vi "Main.vi"(11 "Module Admin":refnum<class "Delacor_lib_QMH_Module Admin.lvclass">) -> ()   [LabVIEW 2024, in "Auto Modo.lvlib"]
doc: "This template is based off of the Queued Message Handler design pattern and the Queued Message Handler project template that ships with LabVIEW.\n\nThe main difference is that the queue is private to this module and communication between modules is performed via Broadcast and Request events.\n\nRequest events are wrapped in public API methods and are handled in the Event Handling Loop (EHL) of this VI. Any module can register for Broadcast events sent by this module. The EHL generates messages based on user interface actions.\n\nThe Message Handling Loop (MHL) processes messages generated by the EHL, or by other messages. The messages are string values, so new messages can be added easily to the Message Cases case structure in the MHL. Each message cluster can also provide an optional value for Message Data, which is a variant that can be converted to whatever message-specific data is required.\n_____\nBased on DQMH Project Template 7.0.1.1316."
uses:
  Auto Modo.lvlib
  <vilib>/Delacor/Delacor QMH/Libraries/Module Admin_class/Delacor_lib_QMH_Module Admin.lvclass
  Sequencer Data Context.ctl
  Sequencer State.ctl
  Module Data--cluster.ctl
  Stop Sequence (Reply Payload)--cluster.ctl
  Start Sequence (Reply Payload)--cluster.ctl
  <vilib>/Delacor/Delacor QMH/Libraries/Message Queue_class/Delacor_lib_QMH_Message Queue.lvclass/Delacor_lib_QMH_Message Queue.ctl
  Stop Argument--cluster.ctl
  <vilib>/Delacor/Delacor QMH/Libraries/Module Admin_class/Delacor_lib_QMH_Module Admin.lvclass/Delacor_lib_QMH_Module Admin.ctl
  Check Idle State Argument--cluster.ctl
  Check Idle State (Reply Payload)--cluster.ctl
  <vilib>/Utility/miscctls.llb/LVPointTypeDef.ctl
  <vilib>/Delacor/Delacor QMH/Libraries/Message Queue_class/Delacor_lib_QMH_Enqueue Message (Single).vi
  <vilib>/Delacor/Delacor QMH/Libraries/Module Admin_class/Delacor_lib_QMH_Get External Launch.vi
  <vilib>/Delacor/Delacor QMH/Libraries/Message Queue_class/Delacor_lib_QMH_Message Queue.lvclass
  Hardware Controller/Hardware Controller.lvlib
  Logger/Logger.lvlib
panel:
  out "Sequencer Data Context":T1={"Sequencer State"=enum."Idle", "Event Timeout"=-1, "Current Index"=0, "Sequence Timeout"=0, "Turbine RPM Array"=[], "Pump RPM Array"=[], "Duration (Seconds) Array"=[], "Folder Path"=path ""}
  out "System State":map{string, dbl}(c390)
  out "error out":errorcluster
  out "Status":string
  in  "Simulate MHL Error":bool
  in  "Simulate EHL Error":bool
  # "Global Variable"
  # "This template is for the DQMH framework. See the block diagram for more information on how to use this template."
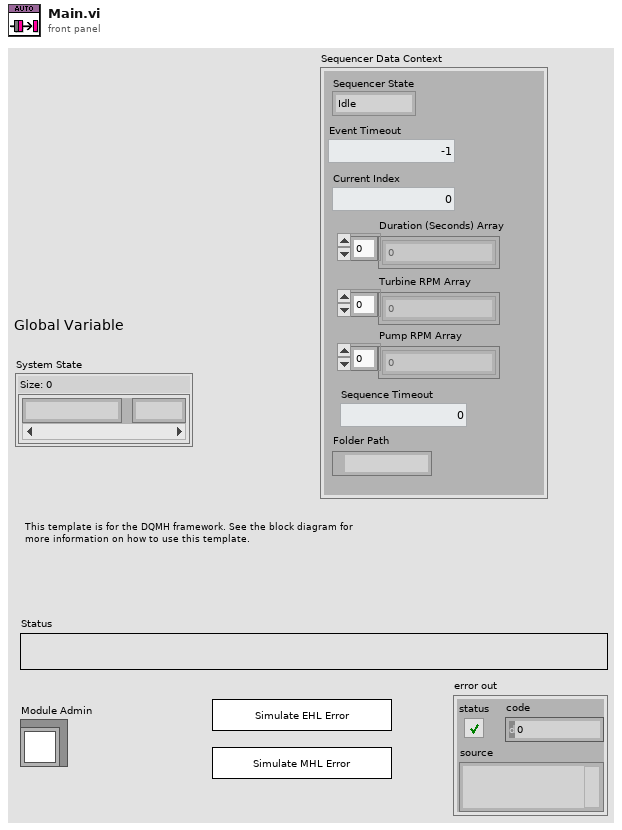
[diagram p1: front panel]
types:
  T1 = typedef "Auto Modo.lvlib/Sequencer Data Context.ctl" = cluster{"Sequencer State":T2, "Event Timeout":i32, "Current Index":i32, "Sequence Timeout":i32, "Turbine RPM Array":dbl[], "Pump RPM Array":dbl[], "Duration (Seconds) Array":dbl[], "Folder Path":path}
  T2 = typedef "Auto Modo.lvlib/Sequencer State.ctl" = enum16{"Idle", "Clear Drive Fault", "Check Drive Fault", "Set Ready to Switch ON", "Check Ready to Switch ON", "Enable Operation", "Check Enable Operation", "Set Drive RPM", "Check Drive RPM", "Next Drive RPM", "Final"}
  T3 = typedef "Auto Modo.lvlib/Request Events--cluster.ctl" = cluster{"Stop Module":refnum<user-event>, "Show Panel":refnum<user-event>, "Hide Panel":refnum<user-event>, "Get Module Execution Status":refnum<user-event>, "Show Diagram":refnum<user-event>, "Start Sequence":refnum<user-event>, "Stop Sequence":refnum<user-event>, "Check Idle State":refnum<user-event>}
  T4 = typedef "Hardware Controller.lvlib/Broadcast Events--cluster.ctl" = cluster{"Module Did Init":refnum<user-event>, "Status Updated":refnum<user-event>, "Error Reported":refnum<user-event>, "Module Did Stop":refnum<user-event>, "Update Module Execution Status":refnum<user-event>, "System State Updated":refnum<user-event>, "EtherCAT Data Updated":refnum<user-event>, "System Fault Updated":refnum<user-event>, "EtherCAT Connection Status Updated":refnum<user-event>, "HardwareController IOLink Data Updated":refnum<user-event>, "IOLink Connection Updated":refnum<user-event>, "HardwareController EtherCAT Data Updated":refnum<user-event>}
  T5 = typedef "Auto Modo.lvlib/Module Data--cluster.ctl" = cluster{"Status":string}
  T6 = typedef "Auto Modo.lvlib/Stop Sequence (Reply Payload)--cluster.ctl" = cluster{"error":errorcluster}
  T7 = typedef "Auto Modo.lvlib/Start Sequence (Reply Payload)--cluster.ctl" = cluster{"error":errorcluster}
  T8 = enum32{"invalid lock state", "Not Locked", "Locked (No Password)", "Password-protected"}
  T9 = typedef "Auto Modo.lvlib/Stop Argument--cluster.ctl" = cluster{"Origin":string, "Exit via Stop Module Req?":bool, "Wait for Module to stop?":bool}
  T10 = typedef "Auto Modo.lvlib/Check Idle State Argument--cluster.ctl" = cluster{"Wait Notifier":refnum<notifier>, "wait for reply":bool}
  T11 = typedef "LVPointTypeDef.ctl" = cluster{"Horizontal":i16, "Vertical":i16}
  T12 = enum32{"Invalid", "Standard", "Closed", "Hidden", "Minimized", "Maximized"}
  T13 = typedef "Auto Modo.lvlib/Check Idle State (Reply Payload)--cluster.ctl" = cluster{"Idle":bool, "error":errorcluster}
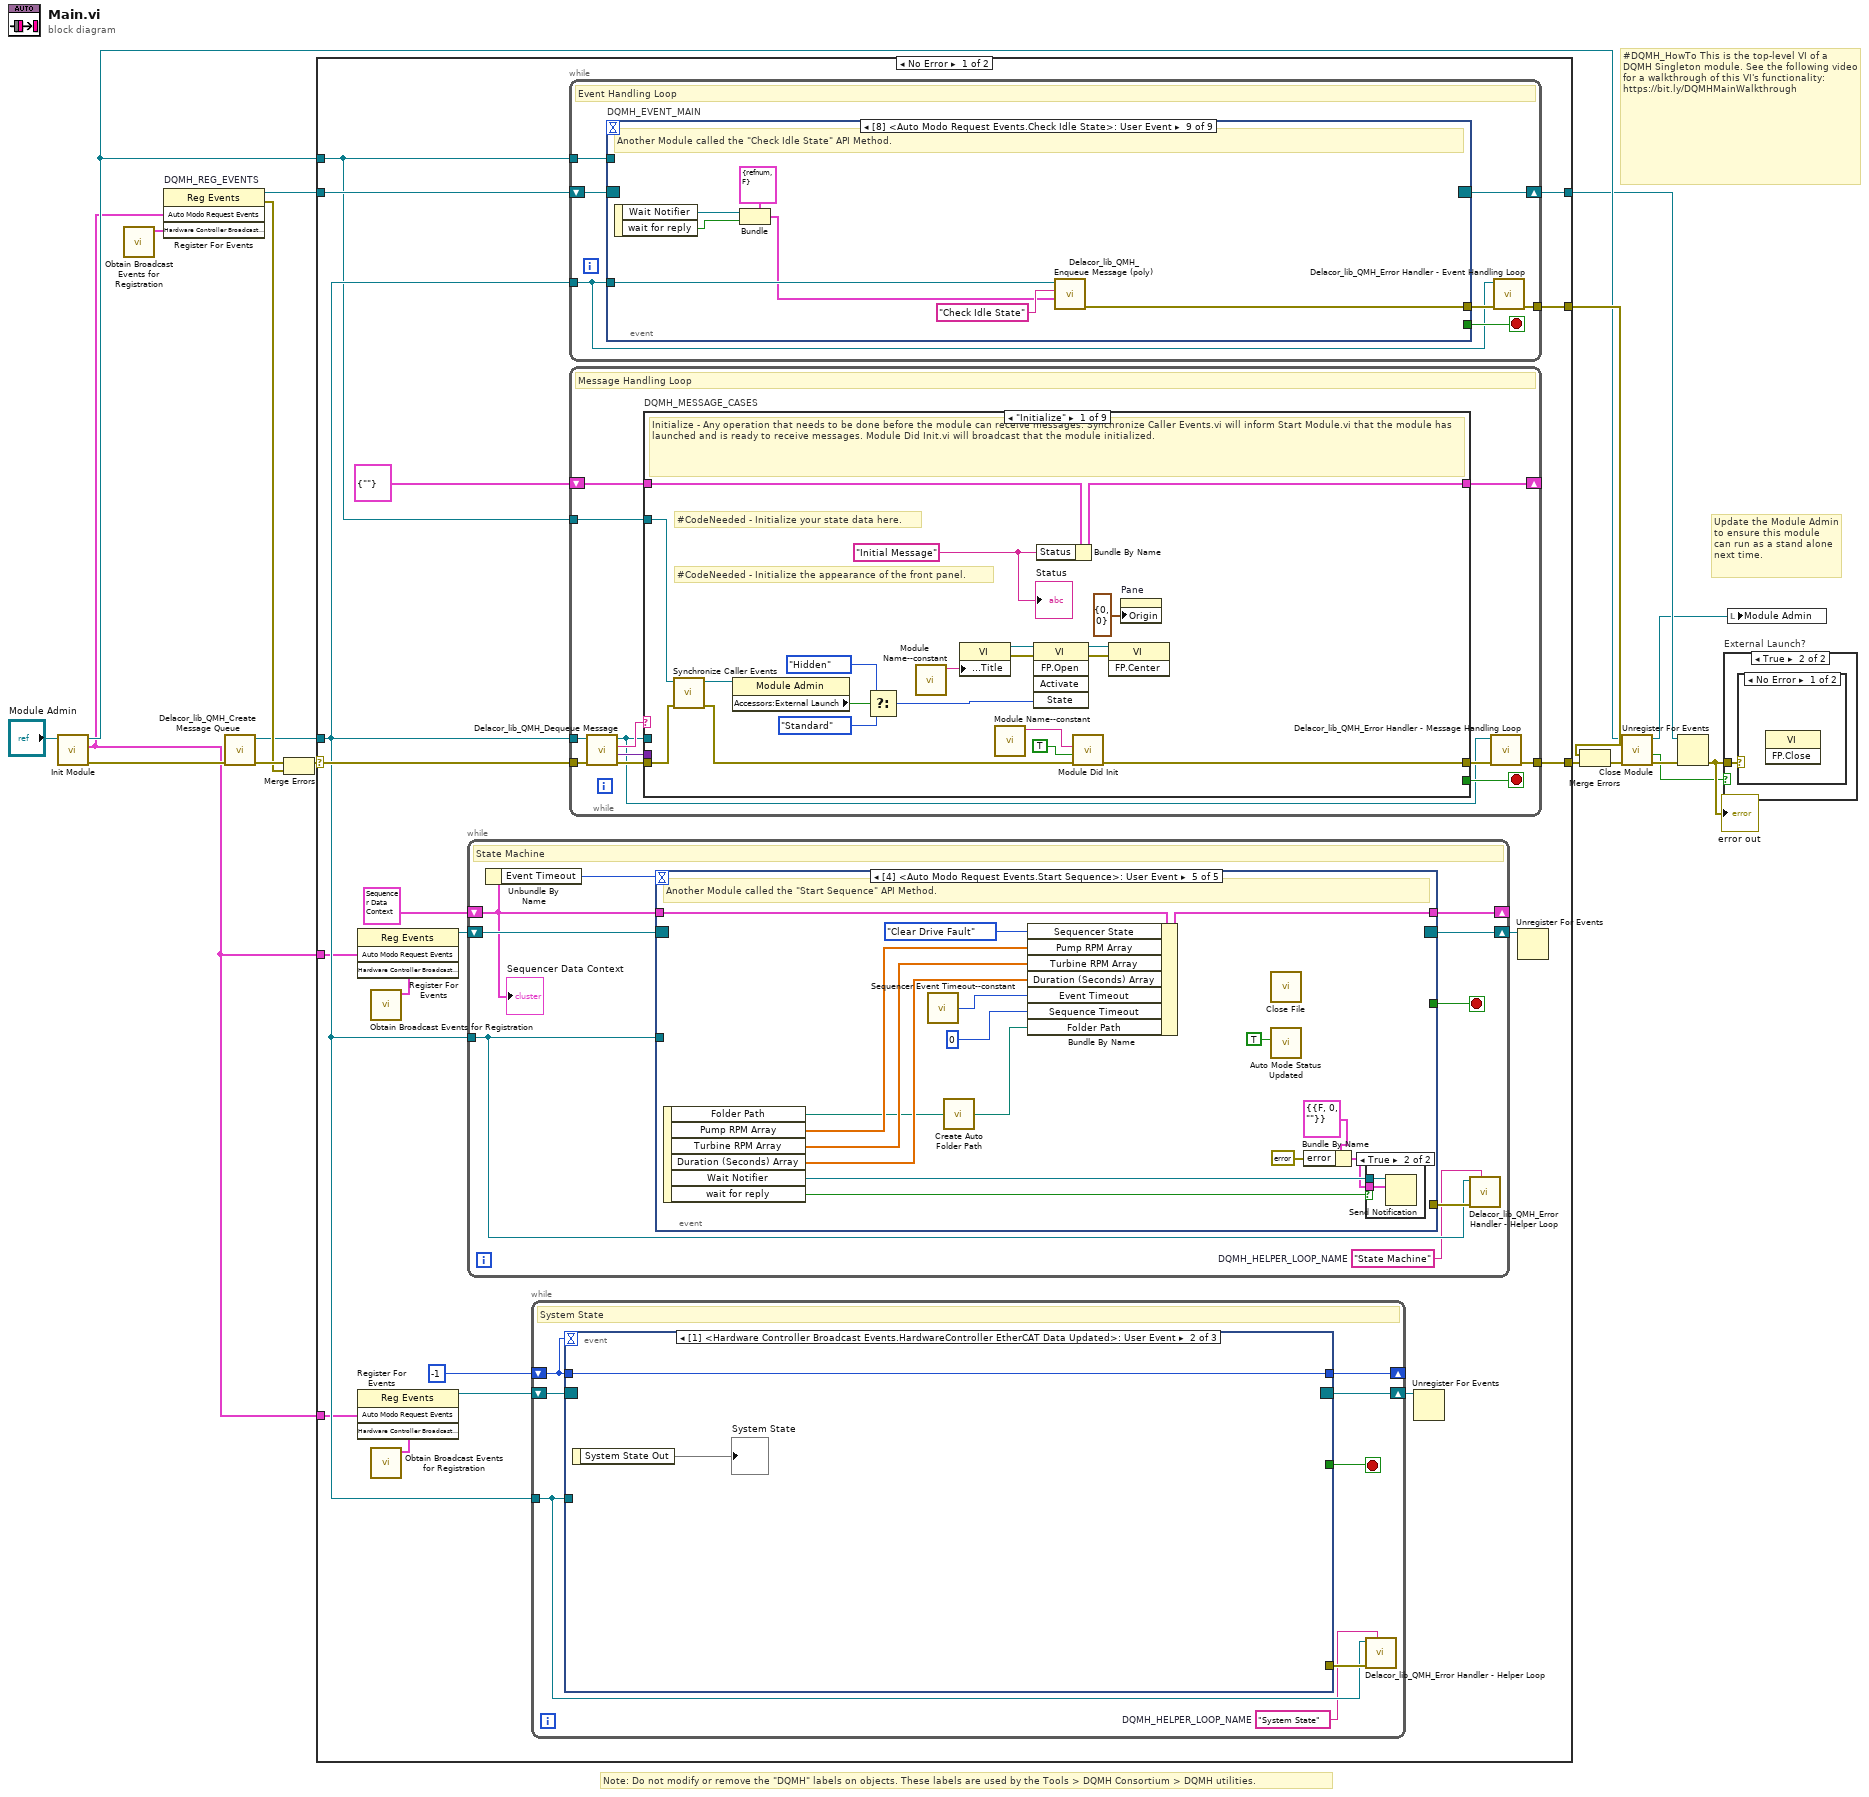
[diagram p0: block diagram]
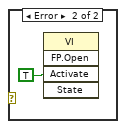
[diagram p3: hidden frame]
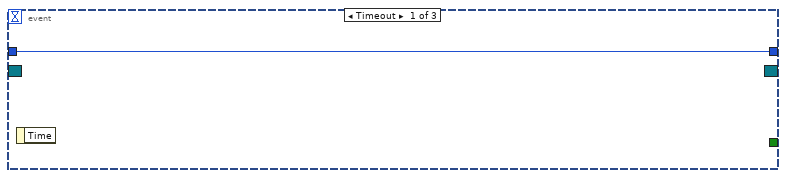
[diagram p4: hidden frame]
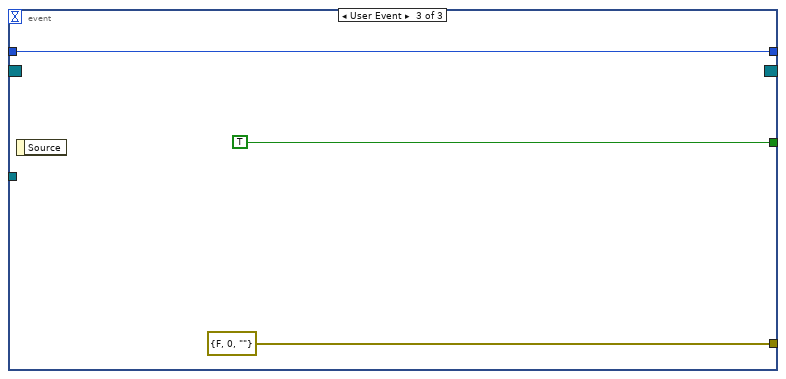
[diagram p5: hidden frame]
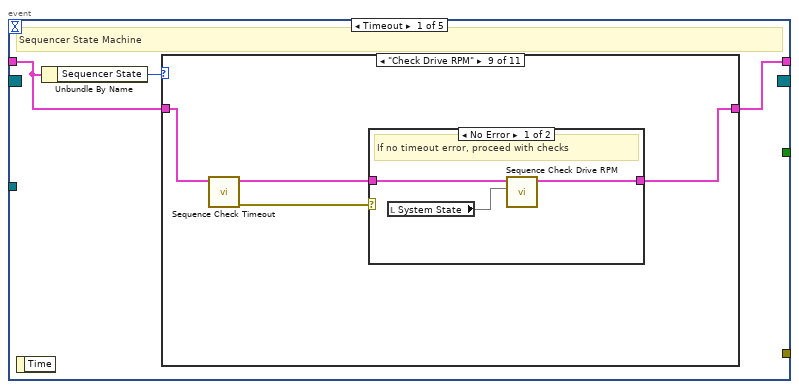
[diagram p6: hidden frame]
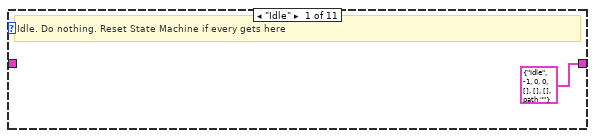
[diagram p7: hidden frame]
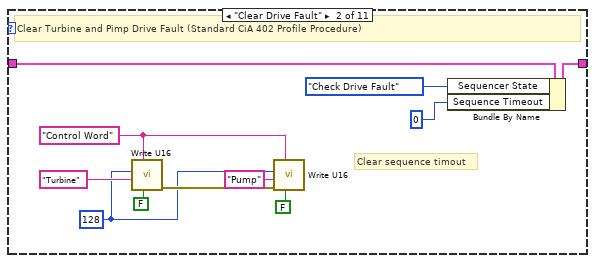
[diagram p8: hidden frame]
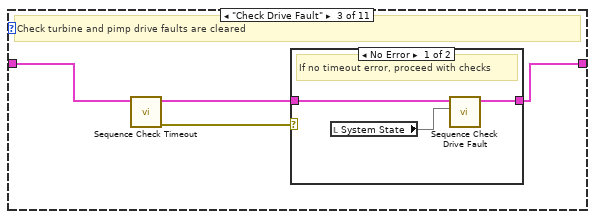
[diagram p9: hidden frame]
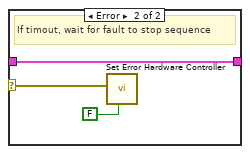
[diagram p10: hidden frame]
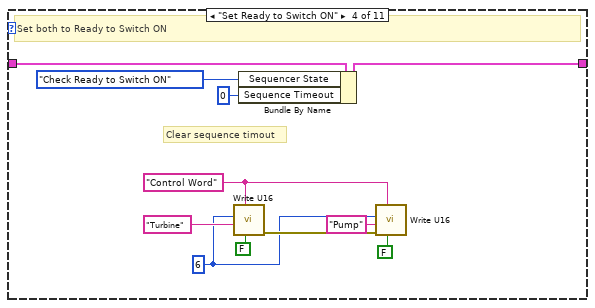
[diagram p11: hidden frame]
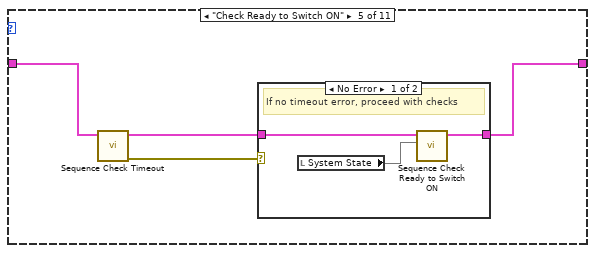
[diagram p12: hidden frame]
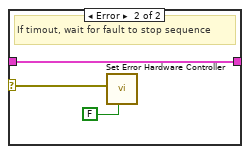
[diagram p13: hidden frame]
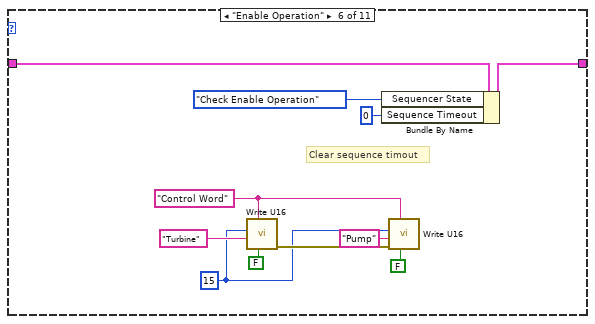
[diagram p14: hidden frame]
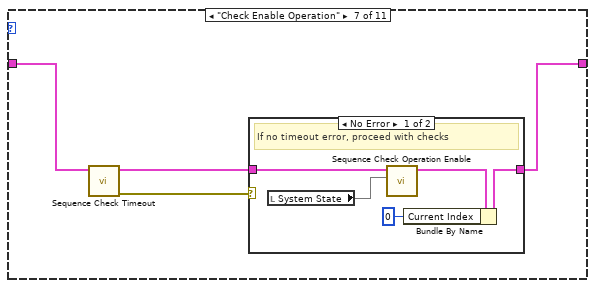
[diagram p15: hidden frame]
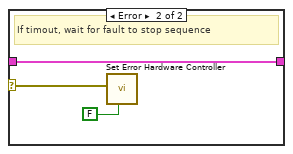
[diagram p16: hidden frame]
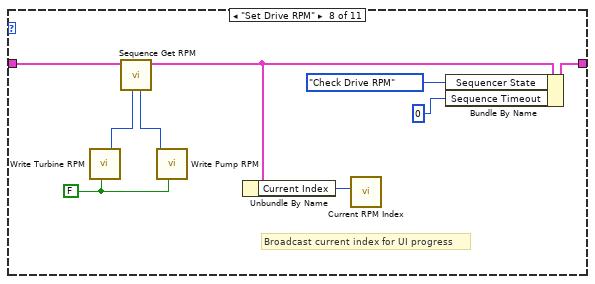
[diagram p17: hidden frame]
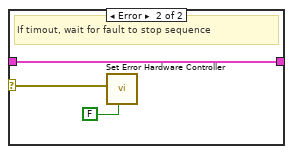
[diagram p18: hidden frame]
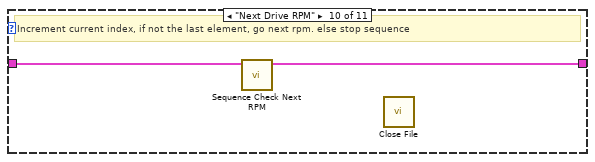
[diagram p19: hidden frame]
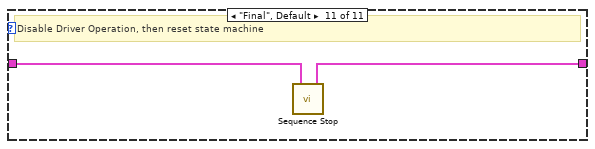
[diagram p20: hidden frame]
diagram:
  # "#DQMH_HowTo This is the top-level VI of a DQMH Singleton module. See the following video for a walkthrough of this VI's functionality: https://bit.ly/DQMHMainWalkthrough"
  # "Note: Do not modify or remove the \"DQMH\" labels on objects. These labels are used by the Tools > DQMH Consortium > DQMH utilities."
  # "Update the Module Admin to ensure this module can run as a stand alone next time."
  n1 = call "Init Module.vi"("Singleton Module Admin in"="Module Admin") -> ("error out"=w17:errorcluster, "Auto Modo Request Events"=w1:T3, "Singleton Module Admin out"=w9:refnum<class "Delacor_lib_QMH_Module Admin.lvclass">)  [unwired: 8 in]
  n2 = call "Obtain Broadcast Events for Registration.vi"() -> ("Hardware Controller Broadcast Events"=w2:T4)  [unwired: 9 in, 2 out]
  n3 = register-events "DQMH_REG_EVENTS"(w1, w2) -> (reference out=w7:refnum<event-registration>, error out=w10:errorcluster)  [unwired: 2 in]
  n4 = call <vilib>:"Delacor_lib_QMH_Create Message Queue.vi"("error in"=w17) -> ("error out"=w12:errorcluster, "Message Queue"=w6:refnum<class "Delacor_lib_QMH_Message Queue.lvclass">)  [unwired: 9 in]
  n5 = Merge Errors(w12, w10) -> (w11:errorcluster)
  n6 = case shown="No Error" w11 {
    selector: w11 -> [w34 w360]
    tunnel: [w36 w359] -> w18
    tunnel: [w33 w358] -> w8
    tunnel: w7 -> [w31 w358]
    tunnel: w6 -> [w30 w353]
    tunnel: [w35 _] -> w15
    tunnel: w9 -> [w29 w354]
    tunnel: w1 -> [w28 _]
    tunnel: w1 -> [w23 _]
    frame No Error {
      n7 = call "Obtain Broadcast Events for Registration.vi"() -> ("Hardware Controller Broadcast Events"=w24:T4)  [unwired: 9 in, 2 out]
      n8 = register-events ("DQMH_HELPER_REGFOREVENTS")(w28, w24) -> (reference out=w26:refnum<event-registration>)  [unwired: 2 in, 1 out]
      n9 = call "Obtain Broadcast Events for Registration.vi"() -> ("Hardware Controller Broadcast Events"=w19:T4)  [unwired: 9 in, 2 out]
      n10 = register-events ("DQMH_HELPER_REGFOREVENTS")(w23, w19) -> (reference out=w21:refnum<event-registration>)  [unwired: 2 in, 1 out]
      n11 = while "DQMH_HELPER_LOOP" {
        shift-right: [w59] -> _
        shift-left: T1 {"Sequencer State"=enum."Clear Drive Fault", "Event Timeout"=-1, "Current Index"=0, "Sequence Timeout"=-1, "Turbine RPM Array"=[], "Pump RPM Array"=[], "Duration (Seconds) Array"=[], "Folder Path"=path ""} ("Sequencer Data Context") -> [w52]
        shift-right: [w57] -> w27
        shift-left: w26 -> [w58]
        tunnel: w30 -> [w54]
        stop <- w56 stop-if-true
        w53 = "State Machine"  # DQMH_HELPER_LOOP_NAME
        # "State Machine"
        n12 = Unbundle By Name(w52) -> ("Event Timeout"=w51:i32)
        n13 = event "DQMH_HELPER_EVENT_STRUCTURE" shown="[4] <Auto Modo Request Events.Start Sequence>: User Event" {
          selector: w58 -> [_ _ _ _ _]
          dyn-events: [_ _ _ _ _] -> w57
          timeout: w51 -> [_ _ _ _ _]
          tunnel: w52 -> [w62 w152 w161 w163 w182]
          tunnel: [w60 w153 w162 w164 w177] -> w59
          tunnel: [_ _ _ TRUE _] -> w56
          tunnel: [_ _ _ errorcluster {"status"=FALSE, "code"=0, "source"=""} ("error constant") _] -> w55
          tunnel: w54 -> [_ _ _ _ _]
          event Timeout {
            # "Sequencer State Machine"
            n14 = event-data() -> ()  [unwired: 1 in, 1 out]
            n15 = Unbundle By Name(w62) -> ("Sequencer State"=w61:T2)
            n16 = case shown="\"Check Drive RPM\"" w61 {
              tunnel: w62 -> [_ w74 w77 w88 w97 w114 w118 w137 w139 w149 w150]
              tunnel: [T1 {"Sequencer State"=enum."Idle", "Event Timeout"=-1, "Current Index"=0, "Sequence Timeout"=0, "Turbine RPM Array"=[], "Pump RPM Array"=[], "Duration (Seconds) Array"=[], "Folder Path"=path ""} ("Sequencer Data Context") w66 w78 w87 w96 w113 w117 w136 w138 w148 w151] -> w60
              frame "Idle" {
                # "Idle. Do nothing. Reset State Machine if every gets here"
              }
              frame "Clear Drive Fault" {
                w73 = "Control Word" ("Variable")
                w68 = u16 128 ("Data")
                # "Clear sequence timout"
                # "Clear Turbine and Pimp Drive Fault (Standard CiA 402 Profile Procedure)"
                n17 = call "Write U16.vi"("wait for reply (T)"=FALSE, "Variable"=w73, "Drive"="Turbine", "Data"=w68) -> ("error out"=w71:errorcluster)  [unwired: 6 in, 1 out]
                n18 = call "Write U16.vi"("wait for reply (T)"=FALSE, "Variable"=w73, "error in"=w71, "Drive"="Pump", "Data"=w68) -> ()  [unwired: 5 in, 2 out]
                n19 = Bundle By Name(cluster=w74, "Sequencer State"=Sequencer_State."Check Drive Fault", "Sequence Timeout"=0) -> (w66:T1)
              }
              frame "Check Drive Fault" {
                # "Check turbine and pimp drive faults are cleared"
                n20 = call "Sequence Check Timeout.vi"("Sequencer Data Context IN"=w77) -> ("error out"=w75:errorcluster, "Sequencer Data Context OUT"=w76:T1)  [unwired: 9 in]
                n21 = case shown="No Error" w75 {
                  selector: w75 -> [_ w82]
                  tunnel: [w81 w84] -> w78
                  tunnel: w76 -> [w79 w84]
                  frame No Error {
                    # "If no timeout error, proceed with checks"
                    n22 = local read "System State"() -> (w80:map{string, dbl})
                    n23 = call "Sequence Check Drive Fault.vi"("System State"=w80, "Sequencer Data Context IN"=w79) -> ("Sequencer Data Context OUT"=w81:T1)  [unwired: 9 in]
                  }
                  frame Error {
                    # "If timout, wait for fault to stop sequence"
                    n24 = call "Set Error Hardware Controller.vi"("wait for reply (T)"=FALSE, "Error Cluster"=w82) -> ()  [unwired: 8 in, 2 out]
                  }
                }
              }
              frame "Set Ready to Switch ON" {
                w95 = "Control Word" ("Variable")
                w90 = u16 6 ("Data")
                # "Clear sequence timout"
                # "Set both to Ready to Switch ON"
                n25 = call "Write U16.vi"("wait for reply (T)"=FALSE, "Variable"=w95, "Drive"="Turbine", "Data"=w90) -> ("error out"=w93:errorcluster)  [unwired: 6 in, 1 out]
                n26 = Bundle By Name(cluster=w88, "Sequencer State"=Sequencer_State."Check Ready to Switch ON", "Sequence Timeout"=0) -> (w87:T1)
                n27 = call "Write U16.vi"("wait for reply (T)"=FALSE, "Variable"=w95, "error in"=w93, "Drive"="Pump", "Data"=w90) -> ()  [unwired: 5 in, 2 out]
              }
              frame "Check Ready to Switch ON" {
                n28 = call "Sequence Check Timeout.vi"("Sequencer Data Context IN"=w97) -> ("error out"=w98:errorcluster, "Sequencer Data Context OUT"=w99:T1)  [unwired: 9 in]
                n29 = case shown="No Error" w98 {
                  selector: w98 -> [_ w103]
                  tunnel: [w102 w105] -> w96
                  tunnel: w99 -> [w100 w105]
                  frame No Error {
                    # "If no timeout error, proceed with checks"
                    n30 = local read "System State"() -> (w101:map{string, dbl})
                    n31 = call "Sequence Check Ready to Switch ON.vi"("System State"=w101, "Sequencer Data Context IN"=w100) -> ("Sequencer Data Context OUT"=w102:T1)  [unwired: 9 in]
                  }
                  frame Error {
                    # "If timout, wait for fault to stop sequence"
                    n32 = call "Set Error Hardware Controller.vi"("wait for reply (T)"=FALSE, "Error Cluster"=w103) -> ()  [unwired: 8 in, 2 out]
                  }
                }
              }
              frame "Enable Operation" {
                w112 = "Control Word" ("Variable")
                w107 = u16 15 ("Data")
                # "Clear sequence timout"
                n33 = call "Write U16.vi"("wait for reply (T)"=FALSE, "Variable"=w112, "Drive"="Turbine", "Data"=w107) -> ("error out"=w110:errorcluster)  [unwired: 6 in, 1 out]
                n34 = Bundle By Name(cluster=w114, "Sequencer State"=Sequencer_State."Check Enable Operation", "Sequence Timeout"=0) -> (w113:T1)
                n35 = call "Write U16.vi"("wait for reply (T)"=FALSE, "Variable"=w112, "error in"=w110, "Drive"="Pump", "Data"=w107) -> ()  [unwired: 5 in, 2 out]
              }
              frame "Check Enable Operation" {
                n36 = call "Sequence Check Timeout.vi"("Sequencer Data Context IN"=w118) -> ("error out"=w119:errorcluster, "Sequencer Data Context OUT"=w120:T1)  [unwired: 9 in]
                n37 = case shown="No Error" w119 {
                  selector: w119 -> [_ w126]
                  tunnel: [w122 w128] -> w117
                  tunnel: w120 -> [w123 w128]
                  frame No Error {
                    # "If no timeout error, proceed with checks"
                    n38 = local read "System State"() -> (w124:map{string, dbl})
                    n39 = call "Sequence Check Operation Enable.vi"("System State"=w124, "Sequencer Data Context IN"=w123) -> ("Sequencer Data Context OUT"=w125:T1)  [unwired: 9 in]
                    n40 = Bundle By Name(cluster=w125, "Current Index"=0) -> (w122:T1)
                  }
                  frame Error {
                    # "If timout, wait for fault to stop sequence"
                    n41 = call "Set Error Hardware Controller.vi"("wait for reply (T)"=FALSE, "Error Cluster"=w126) -> ()  [unwired: 8 in, 2 out]
                  }
                }
              }
              frame "Set Drive RPM" {
                w129 = FALSE ("wait for reply (T)")
                # "Broadcast current index for UI progress"
                n42 = call "Sequence Get RPM.vi"("Sequencer Data Context IN"=w137) -> ("Sequencer Data Context OUT"=w133:T1, "Pump RPM"=w130:i16, "Turbine RPM"=w131:i16)  [unwired: 8 in]
                n43 = call "Write Turbine RPM.vi"("wait for reply (T)"=w129, "RPM"=w131) -> ()  [unwired: 8 in, 2 out]
                n44 = call "Write Pump RPM.vi"("wait for reply (T)"=w129, "RPM"=w130) -> ()  [unwired: 8 in, 2 out]
                n45 = Unbundle By Name(w133) -> ("Current Index"=w132:i32)
                n46 = call "Current RPM Index.vi"("Current Index"=w132) -> ()  [unwired: 10 in, 1 out]
                n47 = Bundle By Name(cluster=w133, "Sequencer State"=Sequencer_State."Check Drive RPM", "Sequence Timeout"=0) -> (w136:T1)
              }
              frame "Check Drive RPM" {
                n48 = call "Sequence Check Timeout.vi"("Sequencer Data Context IN"=w139) -> ("error out"=w140:errorcluster, "Sequencer Data Context OUT"=w141:T1)  [unwired: 9 in]
                n49 = case shown="No Error" w140 {
                  selector: w140 -> [_ w145]
                  tunnel: [w144 w147] -> w138
                  tunnel: w141 -> [w142 w147]
                  frame No Error {
                    # "If no timeout error, proceed with checks"
                    n50 = local read "System State"() -> (w143:map{string, dbl})
                    n51 = call "Sequence Check Drive RPM.vi"("System State"=w143, "Sequencer Data Context IN"=w142) -> ("Sequencer Data Context OUT"=w144:T1)  [unwired: 9 in]
                  }
                  frame Error {
                    # "If timout, wait for fault to stop sequence"
                    n52 = call "Set Error Hardware Controller.vi"("wait for reply (T)"=FALSE, "Error Cluster"=w145) -> ()  [unwired: 8 in, 2 out]
                  }
                }
              }
              frame "Next Drive RPM" {
                # "Increment current index, if not the last element, go next rpm. else stop sequence"
                n53 = call "Sequence Check Next RPM.vi"("Sequencer Data Context IN"=w149) -> ("Sequencer Data Context OUT"=w148:T1)  [unwired: 10 in]
                n54 = call "Close File.vi"() -> ()  [unwired: 9 in, 3 out]
              }
              frame "Final", Default {
                # "Disable Driver Operation, then reset state machine"
                n55 = call "Sequence Stop.vi"("Sequencer Data Context IN"=w150) -> ("Sequencer Data Context OUT"=w151:T1)
              }
            }
          }
          event User Event {
            # "Another Module called the \"Stop Sequence\" API Method."
            n56 = event-data() -> ("Wait Notifier"=w156:refnum<notifier>, "wait for reply"=w155:bool)  [unwired: 1 in]
            n57 = call "Sequence Stop.vi"("Sequencer Data Context IN"=w152) -> ("Sequencer Data Context OUT"=w153:T1)
            n58 = Bundle By Name(cluster=T6 {"error"={"status"=FALSE, "code"=0, "source"=""}} ("Stop Sequence (Reply Payload)"), "error"=errorcluster {"status"=FALSE, "code"=0, "source"=""}) -> (w158:T6)
            n59 = case "DQMH_FIRE_NOTIFIER" shown="True" w155 {
              tunnel: w156 -> [_ w160]
              tunnel: w158 -> [_ w159]
              frame False {
              }
              frame True {
                n60 = Send Notification(notification=w159, notifier=w160) -> ()  [unwired: 1 in, 2 out]
              }
            }
          }
          event User Event {
            n61 = event-data() -> ()  [unwired: 1 in, 1 out]
            n62 = call "Sequence Stop.vi"("Sequencer Data Context IN"=w161) -> ("Sequencer Data Context OUT"=w162:T1)
          }
          event User Event {
            n63 = event-data() -> ()  [unwired: 1 in, 1 out]
            n64 = call "Sequence Stop.vi"("Sequencer Data Context IN"=w163) -> ("Sequencer Data Context OUT"=w164:T1)
          }
          event User Event {
            # "Another Module called the \"Start Sequence\" API Method."
            n65 = event-data() -> ("Folder Path"=w169:path, "Pump RPM Array"=w172:dbl[], "Turbine RPM Array"=w171:dbl[], "Duration (Seconds) Array"=w170:dbl[], "Wait Notifier"=w181:refnum<notifier>, "wait for reply"=w180:bool)  [unwired: 1 in]
            n66 = call "Sequencer Event Timeout--constant.vi"() -> ("Event Timeout (ms)"=w174:i32)  [unwired: 1 in]
            n67 = call "Create Auto Folder Path.vi"("Parent Folder Path"=w169) -> ("Auto Folder Path"=w168:path)
            n68 = Bundle By Name(cluster=w182, "Sequencer State"=Sequencer_State."Clear Drive Fault", "Pump RPM Array"=w172, "Turbine RPM Array"=w171, "Duration (Seconds) Array"=w170, "Event Timeout"=w174, "Sequence Timeout"=0, "Folder Path"=w168) -> (w177:T1)
            n69 = call "Close File.vi"() -> ()  [unwired: 9 in, 3 out]
            n70 = call "Auto Mode Status Updated.vi"("Auto Mode?"=TRUE) -> ()  [unwired: 10 in, 1 out]
            n71 = Bundle By Name(cluster=T7 {"error"={"status"=FALSE, "code"=0, "source"=""}} ("Start Sequence (Reply Payload)"), "error"=errorcluster {"status"=FALSE, "code"=0, "source"=""}) -> (w179:T7)
            n72 = case "DQMH_FIRE_NOTIFIER" shown="True" w180 {
              tunnel: w181 -> [_ w184]
              tunnel: w179 -> [_ w183]
              frame False {
              }
              frame True {
                n73 = Send Notification(notification=w183, notifier=w184) -> ()  [unwired: 1 in, 2 out]
              }
            }
          }
        }
        n74 = call-dynamic "Delacor_lib_QMH_Error Handler - Helper Loop.vi"("Error Debug"=w53, "error in"=w55, "Message Queue in"=w54) -> ()  [unwired: 7 in, 2 out]
        "Sequencer Data Context" <- w52
      }
      n75 = while "DQMH_HELPER_LOOP" {
        shift-right: [w44] -> _
        shift-left: -1 -> [w43]
        shift-right: [w41] -> w22
        shift-left: w21 -> [w42]
        tunnel: w30 -> [w38]
        stop <- w40 stop-if-true
        w37 = "System State"  # DQMH_HELPER_LOOP_NAME
        # "System State"
        n76 = event "DQMH_HELPER_EVENT_STRUCTURE" shown="[1] <Hardware Controller Broadcast Events.HardwareController EtherCAT Data Updated>: User Event" {
          selector: w42 -> [_ _ _]
          dyn-events: [_ _ _] -> w41
          timeout: w43 -> [_ _ _]
          tunnel: w43 -> [w45 w47 w50]
          tunnel: [w45 w47 w50] -> w44
          tunnel: [_ _ TRUE] -> w40
          tunnel: [_ _ errorcluster {"status"=FALSE, "code"=0, "source"=""} ("error constant")] -> w39
          tunnel: w38 -> [_ _ _]
          event Timeout {
            n77 = event-data() -> ()  [unwired: 1 in, 1 out]
          }
          event User Event {
            n78 = event-data() -> ("System State Out"=→"System State":map{string, dbl})  [unwired: 1 in]
          }
          event User Event {
            n79 = event-data() -> ()  [unwired: 1 in, 1 out]
          }
        }
        n80 = call-dynamic "Delacor_lib_QMH_Error Handler - Helper Loop.vi"("Error Debug"=w37, "error in"=w39, "Message Queue in"=w38) -> ()  [unwired: 7 in, 2 out]
      }
      n81 = while {
        tunnel: w30 -> [w185]
        shift-right: [w188] -> w33
        shift-left: w31 -> [w189]
        tunnel: [w190] -> w35
        tunnel: w29 -> [w186]
        stop <- w187 stop-if-true
        # "Event Handling Loop"
        n82 = event "DQMH_EVENT_MAIN" shown="[8] <Auto Modo Request Events.Check Idle State>: User Event" {
          selector: w189 -> [_ _ _ _ _ _ _ _ _]
          dyn-events: [_ _ _ _ _ _ _ _ _] -> w188
          timeout: _ -> [_ _ _ _ _ _ _ _ _]
          tunnel: [_ _ _ _ _ _ TRUE ("Discard?") _ _] -> w187
          tunnel: w185 -> [_ w199 _ _ _ _ w223 w230 w246]
          tunnel: [w197 w200 _ _ w206 _ w226 w232 w240] -> w191
          tunnel: w186 -> [_ _ _ _ _ _ _ w229 _]
          event "Simulate EHL Error": Value Change {
            # "#DQMH_HowTo The 'Simulate EHL Error' button  illustrates how the EHL handles errors. This event is instructional in nature and can be removed."
            # "This case simulates an error being generated by the EHL"
            n83 = event-data() -> ()  [unwired: 1 in, 1 out]
            n84 = call "Module Name--constant.vi"() -> ("Module Name"=w194:string)  [unwired: 11 in]
            n85 = Format Into String(format string="Simulated error originating at Event Handling Loop in %s", w194) -> (resulting string=w195:string)  [unwired: 2 in, 1 out]
            n86 = call <vilib>:"Error Cluster From Error Code.vi"("show call chain? (False)"=TRUE, "error message (\"\")"=w195, "error code (0)"=5000) -> ("error out"=w197:errorcluster)  [unwired: 6 in]
          }
          event "Simulate MHL Error": Value Change {
            # "#DQMH_HowTo The 'Simulate MHL Error' button  illustrates how the MHL handles errors. This event is instructional in nature and can be removed."
            # "This case simulates an error being generated by the MHL"
            n87 = event-data() -> ()  [unwired: 1 in, 1 out]
            n88 = call-poly <vilib>:"Delacor_lib_QMH_Enqueue Message (poly).vi"("Message"="Simulate MHL Error", "Message Queue in"=w199) -> ("error out"=w200:errorcluster)  [unwired: 8 in, 1 out]
          }
          event User Event {
            # "Show the panel of this VI, and send a status updated message to let listeners know."
            # "Another Module called the \"Show Panel\" API Method."
            n89 = event-data() -> ()  [unwired: 1 in, 1 out]
            n90 = control-ref of="This VI"() -> (w202:refnum<vi>)
            n91 = call "Open VI Panel.vi"("VI"=w202) -> ()  [unwired: 10 in, 1 out]
            n92 = call "Status Updated.vi"("Status"="Panel shown." ("format string")) -> ()  [unwired: 10 in, 1 out]
          }
          event User Event {
            # "Hide the panel of this VI, and send a status updated message to let listeners know."
            # "Another Module called the \"Hide Panel\" API Method."
            n93 = event-data() -> ()  [unwired: 1 in, 1 out]
            n94 = control-ref of="This VI"() -> (w204:refnum<vi>)
            n95 = call "Hide VI Panel.vi"("VI"=w204) -> ()  [unwired: 10 in, 1 out]
            n96 = call "Status Updated.vi"("Status"="Panel hidden." ("format string")) -> ()  [unwired: 10 in, 1 out]
          }
          event User Event {
            # "Another Module called the \"Get Module Execution Status\" API Method."
            n97 = event-data() -> ()  [unwired: 1 in, 1 out]
            n98 = call "Update Module Execution Status.vi"("Running?"=TRUE) -> ("error out"=w206:errorcluster)  [unwired: 10 in]
          }
          event User Event {
            # "Another Module called the \"Show Diagram\" API Method. This event is used for debugging."
            n99 = event-data() -> ()  [unwired: 1 in, 1 out]
            n100 = disable-structure shown="RUN_TIME_ENGINE==False" {
              frame condition #0 (active) {
                # "functionality not available in exe"
                n101 = invoke on="Invoke Node" class="VI" method="Lock State.Get"() -> (error out=w212:errorcluster, "Get Lock State"=w211:T8, "pwd in cache"=w208:bool)  [unwired: 4 in, 1 out]
                n102 = Equal?(x=T8."Password-protected", y=w211) -> (x = y?=w209:bool)
                n103 = Compound Arithmetic op=AND(w209, invert w208) -> (w207:bool)
                n104 = case shown="False" w207 {
                  tunnel: w212 -> [w215 _]
                  frame False {
                    n105 = property on="Property Node" class="VI"(error in=w215, "BDWin.Open"=TRUE ("Block Diagram Window:Open")) -> ()  [unwired: 1 in, 2 out]
                    n106 = call "Status Updated.vi"("Status"="Block Diagram shown." ("format string")) -> ()  [unwired: 10 in, 1 out]
                  }
                  frame True {
                    # "Password-protected VI, and the password is not in the cache. Do not show the diagram."
                  }
                }
              }
              frame condition #1 {
              }
            }
          }
          event User Event {
            # "The Stop Module Event can get fired from the Exit message in the MHL. The queue gets destroyed in that case. If the queue no longer exists, the Enqueue Exit as a priority message will return error 1. It is safe to ignore, because the module is already exiting."
            # "Another Module called the \"Stop Module\" API Method  or the Message Handling Loop below."
            n107 = event-data() -> ("Origin"=w222:string, "Exit via Stop Module Req?"=w218:bool, "Wait for Module to stop?"=w217:bool)  [unwired: 1 in]
            n108 = local write "Status"(w222) -> ()
            n109 = Bundle By Name(cluster=T9 {"Origin"="", "Exit via Stop Module Req?"=FALSE, "Wait for Module to stop?"=FALSE} ("Stop Argument"), "Exit via Stop Module Req?"=w218, "Wait for Module to stop?"=w217) -> (w216:T9)
            n110 = call-poly <vilib>:"Delacor_lib_QMH_Enqueue Message (poly).vi"("Priority Message? (F)"=TRUE, "Message Data"=w216, "Message"="Exit", "Message Queue in"=w223) -> ("error out"=w227:errorcluster)  [unwired: 6 in, 1 out]
            n111 = call <vilib>:"Clear Errors.vi"("error in (no error)"=w227, "specific error code to clear (0: all)"=1) -> ("error out"=w226:errorcluster)  [unwired: 4 in, 1 out]
          }
          event Panel Close? {
            w231 = TRUE  # Discard the event, the MHL is responsible for closing and stopping this VI.
            # "Hide the panel or send the 'Exit' message if the user clicks the 'X' on the module main VI panel."
            n112 = event-data() -> ()  [unwired: 1 in, 1 out]
            n113 = property on="Property Node" class="Module Admin"(reference=w229) -> ("Accessors:External Launch"=w228:bool)  [unwired: 1 in, 2 out]
            n114 = case shown="True" w228 {
              tunnel: w230 -> [_ w238]
              tunnel: [_ w239] -> w232
              frame True {
                # "If externally launched, clicking the 'X' hides the panel, but doesn't close it."
                n115 = control-ref of="This VI"() -> (w235:refnum<vi>)
                n116 = call "Hide VI Panel.vi"("VI"=w235) -> ("error out"=w233:errorcluster)  [unwired: 10 in]
                n117 = call "Status Updated.vi"("error in"=w233, "Status"="Panel hidden." ("format string")) -> ()  [unwired: 9 in, 1 out]
              }
              frame False {
                # "If run as a stand-alone VI, clicking the panel 'X' stops the VI."
                n118 = call-poly <vilib>:"Delacor_lib_QMH_Enqueue Message (poly).vi"("Priority Message? (F)"=TRUE, "Message"="Exit", "Message Queue in"=w238) -> ("error out"=w239:errorcluster)  [unwired: 7 in, 1 out]
              }
            }
            n119 = event-data ("Event Filter Node")("Discard?"=w231) -> ()  [unwired: 1 in, 1 out]
          }
          event User Event {
            # "Another Module called the \"Check Idle State\" API Method."
            n120 = event-data() -> ("Wait Notifier"=w242:refnum<notifier>, "wait for reply"=w241:bool)  [unwired: 1 in]
            n121 = Bundle(cluster=T10 {"Wait Notifier"=refnum, "wait for reply"=FALSE} ("Check Idle State Argument"), "Wait Notifier"=w242, "wait for reply"=w241) -> (w243:T10)
            n122 = call-poly <vilib>:"Delacor_lib_QMH_Enqueue Message (poly).vi"("Message Data"=w243, "Message"="Check Idle State", "Message Queue in"=w246) -> ("error out"=w240:errorcluster)  [unwired: 7 in, 1 out]
          }
        }
        n123 = call-dynamic "Delacor_lib_QMH_Error Handler - Event Handling Loop.vi"("error in"=w191, "Message Queue in"=w185) -> ("dup error in"=w190:errorcluster)  [unwired: 8 in, 1 out]
      }
      n124 = while {
        tunnel: w30 -> [w247]
        shift-right: [w255] -> _
        shift-left: T5 {"Status"=""} ("Data Cluster") -> [w256]
        tunnel: w34 -> [w258]
        tunnel: [w250] -> w36
        tunnel: w29 -> [w251]
        stop <- w254 stop-if-true
        # "Message Handling Loop"
        n125 = call-dynamic "Delacor_lib_QMH_Dequeue Message.vi"("error in"=w258, "Message Queue in"=w247) -> ("error out"=w257:errorcluster, "Message Data"=w252:variant, "Message"=w253:string, "Message Queue out"=w248:refnum<class "Delacor_lib_QMH_Message Queue.lvclass">)  [unwired: 6 in]
        n126 = case "DQMH_MESSAGE_CASES" shown="\"Initialize\"" w253 {
          selector: w253 -> [_ _ _ _ _ _ _ _ w348]
          tunnel: w248 -> [_ _ _ _ _ _ w314 w336 _]
          tunnel: w257 -> [w276 w280 w294 w299 w301 w310 w321 w342 w351]
          tunnel: [w274 w280 w292 w298 w301 w309 w317 w337 w352] -> w249
          tunnel: w256 -> [w265 w279 w293 w297 w300 w307 w316 w335 w349]
          tunnel: [w264 w279 w293 w297 w300 w307 w316 w335 w349] -> w255
          tunnel: [_ _ _ _ _ _ _ w334 _] -> w254
          tunnel: w252 -> [_ _ w291 _ _ _ w315 w333 _]
          tunnel: w251 -> [w266 _ _ _ _ _ w313 w328 _]
          frame "Initialize" {
            w260 = "Initial Message" ("Initial Message")
            # "#CodeNeeded - Initialize the appearance of the front panel."
            # "#CodeNeeded - Initialize your state data here."
            # "Initialize - Any operation that needs to be done before the module can receive messages. Synchronize Caller Events.vi will inform Start Module.vi that the module has launched and is ready to receive messages. Module Did Init.vi will broadcast that the module initialized."
            n127 = call "Synchronize Caller Events.vi"("error in"=w276, "Singleton Module Admin in"=w266) -> ("error out"=w275:errorcluster, "Singleton Module Admin out"=w261:refnum<class "Delacor_lib_QMH_Module Admin.lvclass">)  [unwired: 8 in]
            n128 = property on="Property Node" class="Module Admin"(reference=w261) -> ("Accessors:External Launch"=w270:bool)  [unwired: 1 in, 2 out]
            n129 = Select(t=T12."Hidden" ("State"), s=w270, f=T12."Standard" ("State")) -> (s? t:f=w267:T12)
            n130 = call "Module Name--constant.vi"() -> ("Module Name"=w273:string)  [unwired: 11 in]
            n131 = property on="Property Node" class="VI"("Front Panel.Title"=w273) -> (reference out=w272:refnum<vi>, error out=w278:errorcluster)  [unwired: 2 in]
            n132 = call "Module Name--constant.vi"() -> ("Module Name"=w262:string)  [unwired: 11 in]
            n133 = invoke on="Invoke Node" class="VI" method="FP.Open"(reference=w272, error in=w278, "State"=w267) -> (reference out=w271:refnum<vi>, error out=w277:errorcluster)  [unwired: 2 in, 3 out]
            n134 = Bundle By Name(cluster=w265, "Status"=w260) -> (w264:T5)
            n135 = call "Module Did Init.vi"("error in"=w275, "Initialized?"=TRUE, "Origin"=w262) -> ("error out"=w274:errorcluster)  [unwired: 8 in]
            n136 = invoke on="Invoke Node" class="VI" method="FP.Center"(reference=w271, error in=w277) -> ()  [unwired: 1 in, 3 out]
            n137 = property on="Pane" class="Pane"("Origin"=T11 {"Horizontal"=0, "Vertical"=0}) -> ()  [unwired: 2 in, 2 out]
            "Status" <- w260
          }
          frame "---Module Specific---" {
            # "Separator -- The following cases handle messages specific to this Module."
          }
          frame "Check Idle State" {
            # "Ths request return true if current state of sequence is idle."
            n138 = Variant To Data(error in=w294, type=T10 {"Wait Notifier"=refnum, "wait for reply"=FALSE} ("Check Idle State Argument"), Variant=w291) -> (data=w289:T10, error out=w292:errorcluster)
            n139 = Unbundle By Name(w289) -> ("Wait Notifier"=w288:refnum<notifier>, "wait for reply"=w287:bool)
            n140 = local read "Sequencer Data Context"() -> (w284:T1)
            n141 = Unbundle By Name(w284) -> ("Sequencer State"=w283:T2)
            n142 = Equal?(x=w283, y=Sequencer_State."Idle") -> (x = y?=w281:bool)
            n143 = Bundle By Name(cluster=T13 {"Idle"=FALSE, "error"={"status"=FALSE, "code"=0, "source"=""}} ("Check Idle State (Reply Payload)"), "Idle"=w281) -> (w286:T13)
            n144 = case "DQMH_FIRE_NOTIFIER" shown="True" w287 {
              tunnel: w288 -> [_ w296]
              tunnel: w286 -> [_ w295]
              frame False {
              }
              frame True {
                n145 = Send Notification(notification=w295, notifier=w296) -> ()  [unwired: 1 in, 2 out]
              }
            }
          }
          frame "---Copy This Frame---" {
            # "Duplicate this frame when creating new messages.  Change this comment in the duplicated frame to describe this message."
            n146 = Merge Errors(w299) -> (w298:errorcluster)
          }
          frame "---Exit and Error Handling---" {
            # "Separator - The following cases handle errors and exit messages."
          }
          frame "Simulate MHL Error" {
            # "#DQMH_HowTo The 'Simulate MHL Error' button  illustrates how the MHL handles errors. This event is instructional in nature and can be removed."
            # "Simulate an error occurring at the MHL"
            n147 = call "Module Name--constant.vi"() -> ("Module Name"=w303:string)  [unwired: 11 in]
            n148 = Format Into String(format string="Simulated error originating at Message Handling Loop in %s", w303) -> (resulting string=w304:string)  [unwired: 2 in, 1 out]
            n149 = call <vilib>:"Error Cluster From Error Code.vi"("show call chain? (False)"=TRUE, "error message (\"\")"=w304, "error code (0)"=5001) -> ("error out"=w308:errorcluster)  [unwired: 6 in]
            n150 = Merge Errors(w310, w308) -> (w309:errorcluster)
          }
          frame "Error" {
            # "#CodeRecommended - If the module is running in standalone mode (External Launch = FALSE), this code will pop up an error dialog and call the 'Exit' message if an error occurs. Add more fine-grained error management here."
            # "Error - Check the error message data and respond accordingly. This message is sent by the \"Error Handler\" VIs at the end of each loop in this application."
            n151 = property on="Property Node" class="Module Admin"(reference=w313) -> ("Accessors:External Launch"=w312:bool)  [unwired: 1 in, 2 out]
            n152 = Variant To Data(error in=w321, type=errorcluster {"status"=FALSE, "code"=0, "source"=""} ("error constant"), Variant=w315) -> (data=w311:errorcluster, error out=w319:errorcluster)
            n153 = local write "error out"(w311) -> ()
            n154 = call "Error Reported.vi"("Error"=w311) -> ()  [unwired: 10 in, 1 out]
            n155 = case shown="False" w312 {
              tunnel: [w326 _] -> w318
              tunnel: w314 -> [w324 _]
              tunnel: w311 -> [w325 _]
              frame False {
                n156 = disable-structure shown="Default" {
                  disable-tunnel: w325 -> [w327 _]
                  frame condition #0 (active) {
                    # "If the module is running standalone, then pop up an error dialog and call the \"Exit\" message."
                    n157 = call <vilib>:"Simple Error Handler.vi"("error in (no error)"=w327) -> ()  [unwired: 4 in, 5 out]
                  }
                  frame condition #1 {
                    # "To prevent the Simple Error Handler VI from being loaded (e.g. when deploying to a Real-Time target), add the Conditional Disable Symbol \"DQMH_Disable_SEH\" to your project and set it to TRUE."
                  }
                }
                n158 = call-poly <vilib>:"Delacor_lib_QMH_Enqueue Message (poly).vi"("Priority Message? (F)"=TRUE, "Message"="Exit", "Message Queue in"=w324) -> ("error out"=w326:errorcluster)  [unwired: 7 in, 1 out]
              }
              frame True {
                # "If the module was launched externally, calling the Error Reported broadcast VI is the only action performed by the \"Error\" message. The module's caller can then process the error appropriately."
              }
            }
            n159 = Merge Errors(w319, w318) -> (w317:errorcluster)
          }
          frame "Exit" {
            w332 = 91  # 91: not all Exit messages will have an argument
            w334 = TRUE  # Stop the VI
            # "Release the message queue reference"
            # "#CodeNeeded - Add any required cleanup code here."
            # "Exit - Exit the application."
            n160 = Variant To Data(error in=w342, type=T9 {"Origin"="", "Exit via Stop Module Req?"=FALSE, "Wait for Module to stop?"=FALSE} ("Stop Argument"), Variant=w333) -> (data=w330:T9, error out=w339:errorcluster)
            n161 = call <vilib>:"Clear Errors.vi"("error in (no error)"=w339, "specific error code to clear (0: all)"=w332) -> ("error out"=w341:errorcluster)  [unwired: 4 in, 1 out]
            n162 = control-ref of="This VI"() -> (w329:refnum<vi>)
            n163 = call-dynamic "Delacor_lib_QMH_Release Message Queue.vi"("error in"=w341, "Message Queue"=w336) -> ("error out"=w340:errorcluster)  [unwired: 9 in]
            n164 = call "Handle Exit.vi"("Stop Argument"=w330, "Admin in"=w328, "VI reference"=w329) -> ("error out"=w338:errorcluster)  [unwired: 7 in, 1 out]
            n165 = Merge Errors(w340, w338) -> (w337:errorcluster)
            n166 = call "Error Reported.vi"("Error"=w337) -> ()  [unwired: 10 in, 1 out]
          }
          frame Default {
            # "'Default' case only runs if there is a message that isn't defined in any of the other cases.  Output a programming error."
            n167 = call "Module Name--constant.vi"() -> ("Module Name"=w347:string)  [unwired: 11 in]
            n168 = Format Into String(format string="The invalid message string \"%s\" was received in the Message Handling Loop for module \"%s\".", w348, w347) -> (resulting string=w343:string)  [unwired: 2 in, 1 out]
            n169 = call <vilib>:"Error Cluster From Error Code.vi"("show call chain? (False)"=TRUE, "error message (\"\")"=w343, "error code (0)"=1) -> ("error out"=w350:errorcluster)  [unwired: 6 in]
            n170 = Merge Errors(w351, w350) -> (w352:errorcluster)
          }
        }
        n171 = call-dynamic "Delacor_lib_QMH_Error Handler - Message Handling Loop.vi"("error in"=w249, "Message Queue in"=w248) -> ("dup error in"=w250:errorcluster)  [unwired: 8 in, 1 out]
      }
      n172 = Unregister For Events(event registration refnum=w22) -> ()  [unwired: 1 in, 1 out]
      n173 = Unregister For Events(event registration refnum=w27) -> ()  [unwired: 1 in, 1 out]
    }
    frame Error {
      # "Synchronize Caller Events.vi will inform Start Module.vi that the module has launched and will let the code calling Start Module.vi register for broadcasts and would permit the caller receive the broadcast that an error occurred at launch time."
      n174 = call-dynamic "Delacor_lib_QMH_Release Message Queue.vi"("error in"=w360, "Message Queue"=w353) -> ("error out"=w359:errorcluster)  [unwired: 9 in]
      n175 = call "Synchronize Caller Events.vi"("Singleton Module Admin in"=w354) -> ("error out"=w361:errorcluster)  [unwired: 9 in, 1 out]
      n176 = call "Module Name--constant.vi"() -> ("Module Name"=w357:string)  [unwired: 11 in]
      n177 = Format Into String(format string="An error occurred during initialization. %s is no longer running.", w357) -> (resulting string=w355:string)  [unwired: 2 in, 1 out]
      n178 = Merge Errors(w359, w361) -> (w362:errorcluster)
      n179 = call "Error Reported.vi"("Additional Information"=w355, "Error"=w362) -> ()  [unwired: 9 in, 1 out]
    }
  }
  n180 = Merge Errors(w15, w18) -> (w14:errorcluster)
  n181 = call "Close Module.vi"("error in"=w14, "Module Admin in"=w9) -> ("error out"=w16:errorcluster, "External Launch"=w3:bool, "Module Admin out"=w4:refnum<class "Delacor_lib_QMH_Module Admin.lvclass">)  [unwired: 7 in]
  n182 = Unregister For Events(event registration refnum=w8, error in=w16) -> (error out=w13:errorcluster)
  "error out" <- w13
  n183 = case "External Launch?" shown="True" w3 {
    tunnel: w13 -> [_ w363]
    frame False {
    }
    frame True {
      n184 = case shown="No Error" w363 {
        frame No Error {
          n185 = invoke on="Invoke Node" class="VI" method="FP.Close"() -> ()  [unwired: 3 in, 3 out]
        }
        frame Error {
          n186 = invoke on="Invoke Node" class="VI" method="FP.Open"("Activate"=TRUE ("Activate?")) -> ()  [unwired: 4 in, 5 out]
        }
      }
    }
  }
  n187 = local write "Module Admin"(w4) -> ()
